vi "GuardaMordasses.vi"(8 "error out":errorcluster, 10 "Mordasses":T1(array[cluster]) {"ID_M" items=["Nº1", "Nº2", "Nº4", "Nº8", "Nº9", "Nº11", "Nº12", "CUERNO_CAZA", "DEF_USER_1", "DEF_USER_2", "DEF_USER_3", "DEF_USER_4", "NO_PRESENTE"]}, 11 "Clau":string) -> (2 "NMordasses":string)   [LabVIEW 2017]
uses:
  <vilib>/registry/registry.llb/Registry RtKey.ctl
  <vilib>/registry/registry.llb/Write Registry Value Simple STR.vi
panel:
  out "ID_M 2":u16(ring) items=["Nº1", "Nº2", "Nº4", "Nº8", "Nº9", "Nº11", "Nº12", "CUERNO_CAZA", "DEF_USER_1", "DEF_USER_2", "DEF_USER_3", "DEF_USER_4", "NO_PRESENTE"]
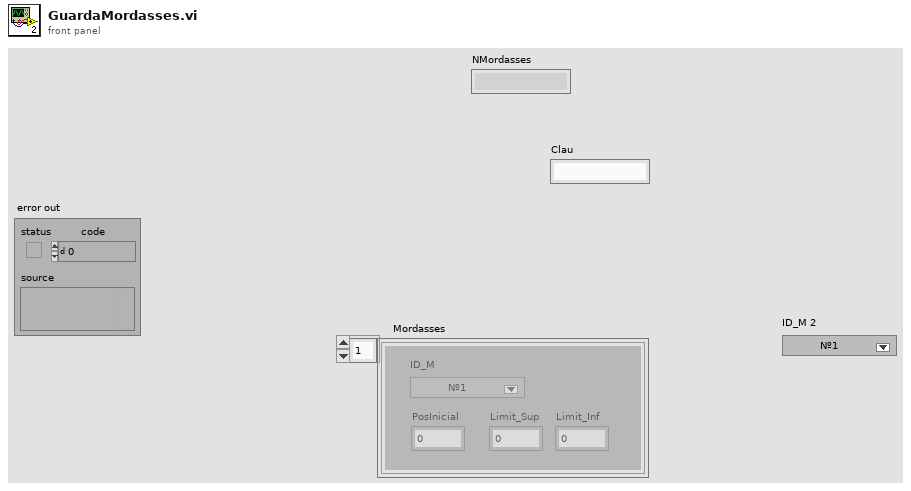
[diagram p1: front panel]
types:
  T1 = cluster{"ID_M":u16, "PosInicial":dbl, "Limit_Sup":dbl, "Limit_Inf":dbl}[]
  T2 = typedef "Registry RtKey.ctl" = enum32{"HKEY_CLASSES_ROOT", "HKEY_CURRENT_USER", "HKEY_LOCAL_MACHINE", "HKEY_USERS", "HKEY_PERFORMANCE_DATA", "HKEY_CURRENT_CONFIG", "HKEY_DYN_DATA"}
  T3 = typedef "Registry refnum.ctl" = refnum<k1>
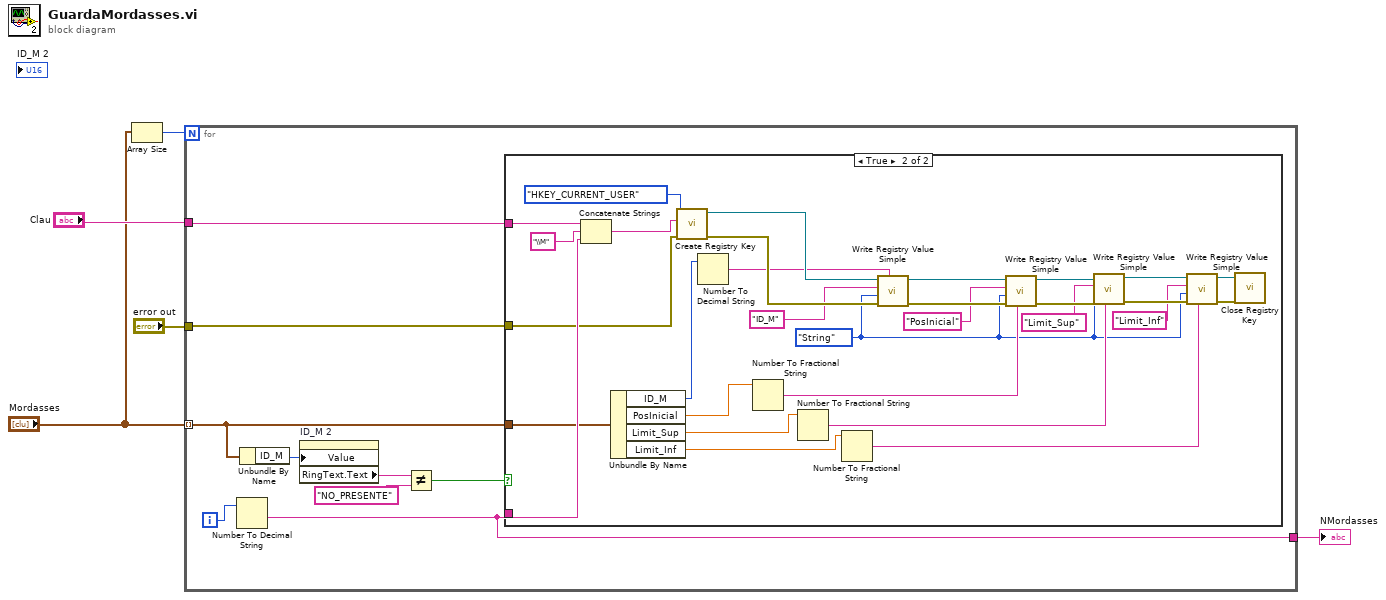
[diagram p0: block diagram]
diagram:
  n1 = Array Size(array="Mordasses") -> (size(s)=w1:i32)
  n2 = for {
    N: w1 -> [_]
    tunnel: "Mordasses" -> [w12] mode=indexing
    tunnel: "error out" -> [w13]
    tunnel: "Clau" -> [w14]
    tunnel: [w8] -> w3
    i -> [w7]
    n3 = Number To Decimal String(number=w7) -> (decimal integer string=w8:string)  [unwired: 1 in]
    n4 = Unbundle By Name(w12) -> ("ID_M"=w11:u16)
    n5 = property on="ID_M 2" class="Ring (strict)"("Value"=w11) -> ("RingText.Text"=w10:string)  [unwired: 2 in, 2 out]
    n6 = Not Equal?(x=w10, y="NO_PRESENTE") -> (x != y?=w6:bool)
    n7 = case shown="True" w6 {
      tunnel: w14 -> [_ w44]
      tunnel: w8 -> [_ w43]
      tunnel: w13 -> [_ w16]
      tunnel: w12 -> [_ w15]
      frame False {
      }
      frame True {
        w17 = enum16{"String", "Binary", "DWORD"}."String" ("simple data type")
        n8 = Concatenate Strings(w44, "\\M" ("string"), w43) -> (w40:string)
        n9 = Unbundle By Name(w15) -> ("ID_M"=w37:u16, "PosInicial"=w31:dbl, "Limit_Sup"=w29:dbl, "Limit_Inf"=w21:dbl)
        n10 = call <vilib>:"Create Registry Key.vi"("error in (no error)"=w16, "subkey"=w40, "root key (HKEY_LOCAL_MACHINE)"=Registry_RtKey."HKEY_CURRENT_USER") -> ("error out"=w38:errorcluster, "refnum out"=w39:T3)  [unwired: 6 in, 1 out]
        n11 = Number To Decimal String(number=w37) -> (decimal integer string=w36:string)  [unwired: 1 in]
        n12 = Number To Fractional String(number=w31) -> (F-format string=w30:string)  [unwired: 3 in]
        n13 = Number To Fractional String(number=w29) -> (F-format string=w25:string)  [unwired: 3 in]
        n14 = Number To Fractional String(number=w21) -> (F-format string=w20:string)  [unwired: 3 in]
        n15 = call-poly <vilib>:"Write Registry Value Simple.vi"("String/Binary data"=w36, "error in (no error)"=w38, "simple data type"=w17, "value"="ID_M", "refnum"=w39) -> ("error out"=w34:errorcluster, "refnum out"=w33:T3)  [unwired: 3 in]
        n16 = call-poly <vilib>:"Write Registry Value Simple.vi"("String/Binary data"=w30, "error in (no error)"=w34, "simple data type"=w17, "value"="PosInicial", "refnum"=w33) -> ("error out"=w27:errorcluster, "refnum out"=w28:T3)  [unwired: 3 in]
        n17 = call-poly <vilib>:"Write Registry Value Simple.vi"("String/Binary data"=w25, "error in (no error)"=w27, "simple data type"=w17, "value"="Limit_Sup", "refnum"=w28) -> ("error out"=w23:errorcluster, "refnum out"=w24:T3)  [unwired: 3 in]
        n18 = call-poly <vilib>:"Write Registry Value Simple.vi"("String/Binary data"=w20, "error in (no error)"=w23, "simple data type"=w17, "value"="Limit_Inf", "refnum"=w24) -> ("error out"=w18:errorcluster, "refnum out"=w19:T3)  [unwired: 3 in]
        n19 = call <vilib>:"Close Registry Key.vi"("error in (no error)"=w18, "refnum"=w19) -> ()  [unwired: 5 in, 1 out]
      }
    }
  }
  "NMordasses" <- w3
